vi "PixelFly_Status_FG.vi"(9 "stop":bool, 10 "Action":enum16{"Write", "Read"}(ring)) -> (1 "stopped":bool)   [LabVIEW 2009, in "Hardware.lvlib" / "Channels.lvlib"]
uses:
  Channels.lvlib
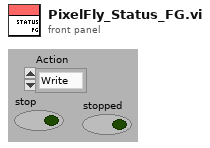
[diagram p1: front panel]
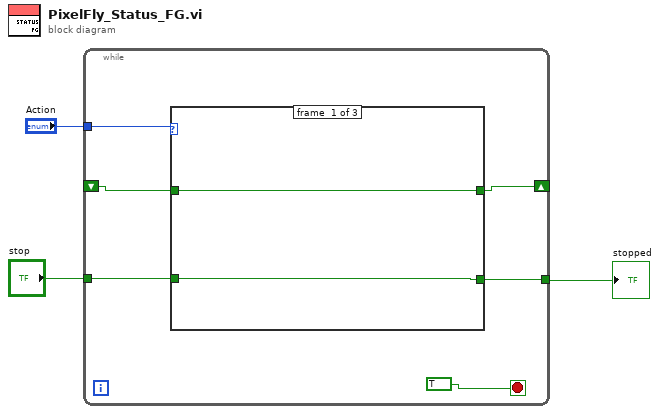
[diagram p0: block diagram]
diagram:
  n1 = while {
    tunnel: "Action" -> [w9]
    shift-right: [w5] -> _
    shift-left: _ -> [w7]
    tunnel: [w6] -> w1
    tunnel: "stop" -> [w4]
    stop <- TRUE stop-if-true
    n2 = case shown="\"Write\"" w9 {
      tunnel: [w11 w12 w13] -> w5
      tunnel: w4 -> [w10 w12 _]
      tunnel: w7 -> [w11 _ w13]
      tunnel: [w10 w12 w13] -> w6
      frame #0 {
      }
      frame #1 {
      }
      frame #2 {
      }
    }
  }
  "stopped" <- w1
